vi "From.vi"(1 "Value":string) -> (0 "String":refnum<class "String.lvclass">)   [LabVIEW 2018, in "Toolkit.lvlib" / "Data.lvlib" / "String.lvclass"]
uses:
  String.lvclass
  String.lvclass/String.ctl
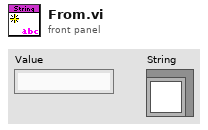
[diagram p1: front panel]
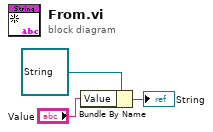
[diagram p0: block diagram]
diagram:
  n1 = Bundle By Name(cluster=refnum<class "String.lvclass"> refnum ("Toolkit.lvlib:Data.lvlib:String.lvclass"), "Value"="Value") -> (→"String":refnum<class "String.lvclass">)
